vi "Initiate Acquisition.vi"(8 "error in":errorcluster, 11 "FPGA VI Reference In":refnum<k20>) -> (0 "error out":errorcluster, 3 "FPGA VI Reference Out":refnum<k20>)   [LabVIEW 2012, in "FlexRIO Host Library (User).lvlib"]
doc: "This start acquisition by switching OFF and ON \"Arm Acquire button\".\nThis VI also starts DMA FIFO."
uses:
  <userlib>/FlexRIO Host Library/FlexRIO Host Library (User).lvlib
  <vilib>/rvi/interface/nirviReadWriteControl/nirviReadWriteControl.xnode
  NiFpgaLv.dll
  <vilib>/Utility/error.llb/Error Cluster From Error Code.vi
  <vilib>/rvi/interface/Simulation/niFpgaSimulationCallBeginRW.vi
  <vilib>/rvi/errors/niLvFpgaAdjustHostInterfaceError.vi
panel:
  out "Current State":T1(ring)
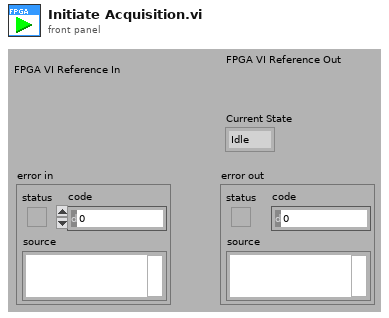
[diagram p1: front panel]
types:
  T1 = enum8{"Idle", "Arm Acquisition Engine", "Acquire Pre-Trigger Samples", "Wait for Trigger", "Acquisition Hold Off Time", "Read Data from Buffer", "Check Records Done?", "Re-Arm State", "Flush Available Data"}
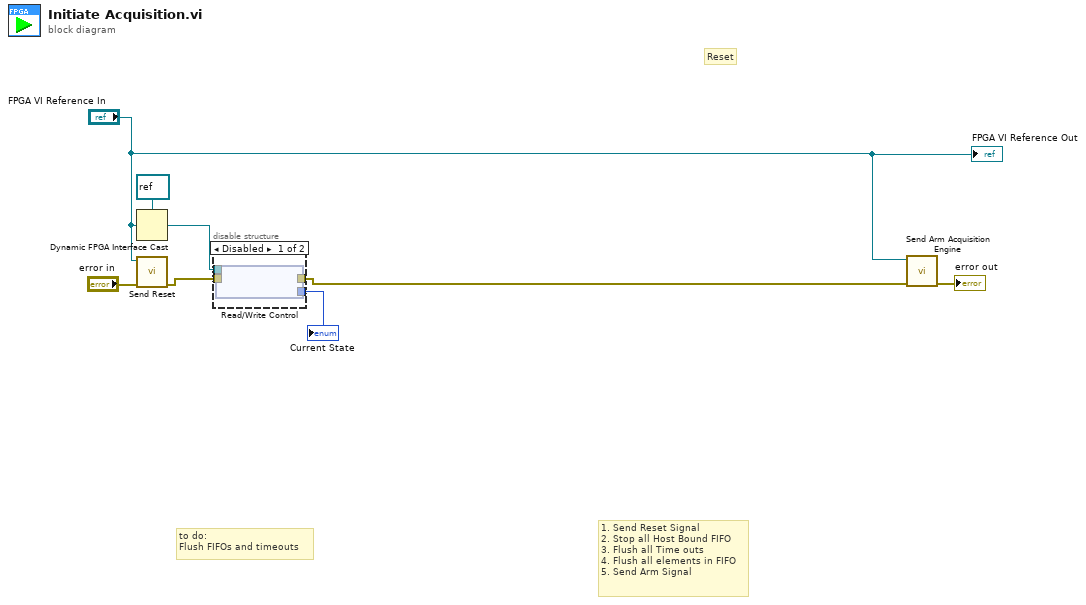
[diagram p0: block diagram]
diagram:
  # "Reset"
  # "to do:\nFlush FIFOs and timeouts"
  # "1. Send Reset Signal\n2. Stop all Host Bound FIFO\n3. Flush all Time outs\n4. Flush all elements in FIFO\n5. Send Arm Signal"
  n1 = Dynamic FPGA Interface Cast(Session In=refnum<k20> refnum ("Type"), Type="FPGA VI Reference In") -> (Session Out=w4:refnum<k20>)
  n2 = call <userlib>:"Send Reset.vi"("error in"="error in", "FPGA VI Reference In"="FPGA VI Reference In") -> ("error out"=w5:errorcluster)  [unwired: 8 in, 1 out]
  n3 = disable-structure shown="Disabled" {
    disable-tunnel: w5 -> [w12 w13]
    disable-tunnel: w4 -> [w11 _]
    disable-tunnel: [w10 w13] -> w3
    disable-tunnel: [w9 _] -> w2
    frame Disabled {
      n4 = xnode "Read/Write Control"("FPGA VI Reference In"=w11, "error in"=w12) -> ("error out"=w10:errorcluster, "Current State"=w9:T1)  [unwired: 1 out]
    }
    frame Enabled {
    }
  }
  "Current State" <- w2
  n5 = call <userlib>:"Send Arm Acquisition Engine.vi"("error in"=w3, "FPGA VI Reference In"="FPGA VI Reference In") -> ("error out"=→"error out":errorcluster)  [unwired: 8 in, 1 out]
  "FPGA VI Reference Out" <- "FPGA VI Reference In"
